vi "Get String Data.vi"(8 "error in (no error)":errorcluster, 11 "Data in":string) -> (0 "error out":errorcluster, 2 "String":string, 3 "Data out":string)   [LabVIEW 2013, in "Hierarchy Framework.lvlib" / "Section.lvclass"]
uses:
  Section.lvclass
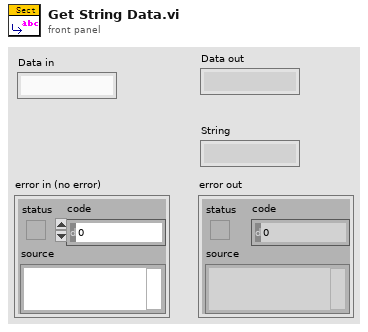
[diagram p1: front panel]
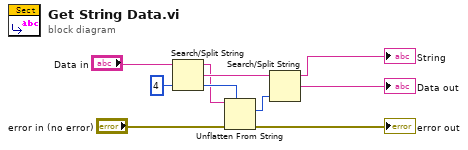
[diagram p0: block diagram]
diagram:
  n1 = Search/Split String(string="Data in", offset (0)=4 ("偏移量(0)")) -> (substring before match=w5:string, match + rest of string=w7:string, offset of match=w6:i32)  [unwired: 1 in]
  n2 = Unflatten From String(type=w6, binary string=w5, error in (no error)="error in (no error)") -> (value=w8:i32, error out=→"error out":errorcluster)  [unwired: 2 in, 1 out]
  n3 = Search/Split String(string=w7, offset (0)=w8) -> (substring before match=→"String":string, match + rest of string=→"Data out":string)  [unwired: 1 in, 1 out]
